vi "PCO_GetTimingStruct.vi"(8 "error in (no error)":errorcluster {"code" format="%x"}, 11 "ph":u64) -> (0 "error out":errorcluster {"code" format="%x"}, 1 "strTiming":T1, 2 "ErrorMessage":i32 format="%x", 3 "ph out":u64)   [LabVIEW 2019, in "SDK.lvlib" / "TimingControl.lvlib"]
doc: "<b>Description:</b>\nTiming related information is queried from the camera and the variables of the PCO_Timing structure are filled with this information. This function is a combined version of the functions which request information about the current settings of timing related parameter. For a detailed description of each parameter see the functions in this chapter.\n\n<b>Supported camera type:</b>\nAll cameras\n\n<b>Descriptor dependency:</b>\nNone"
uses:
  TimingControl.lvlib
  Structures/Structures.lvlib
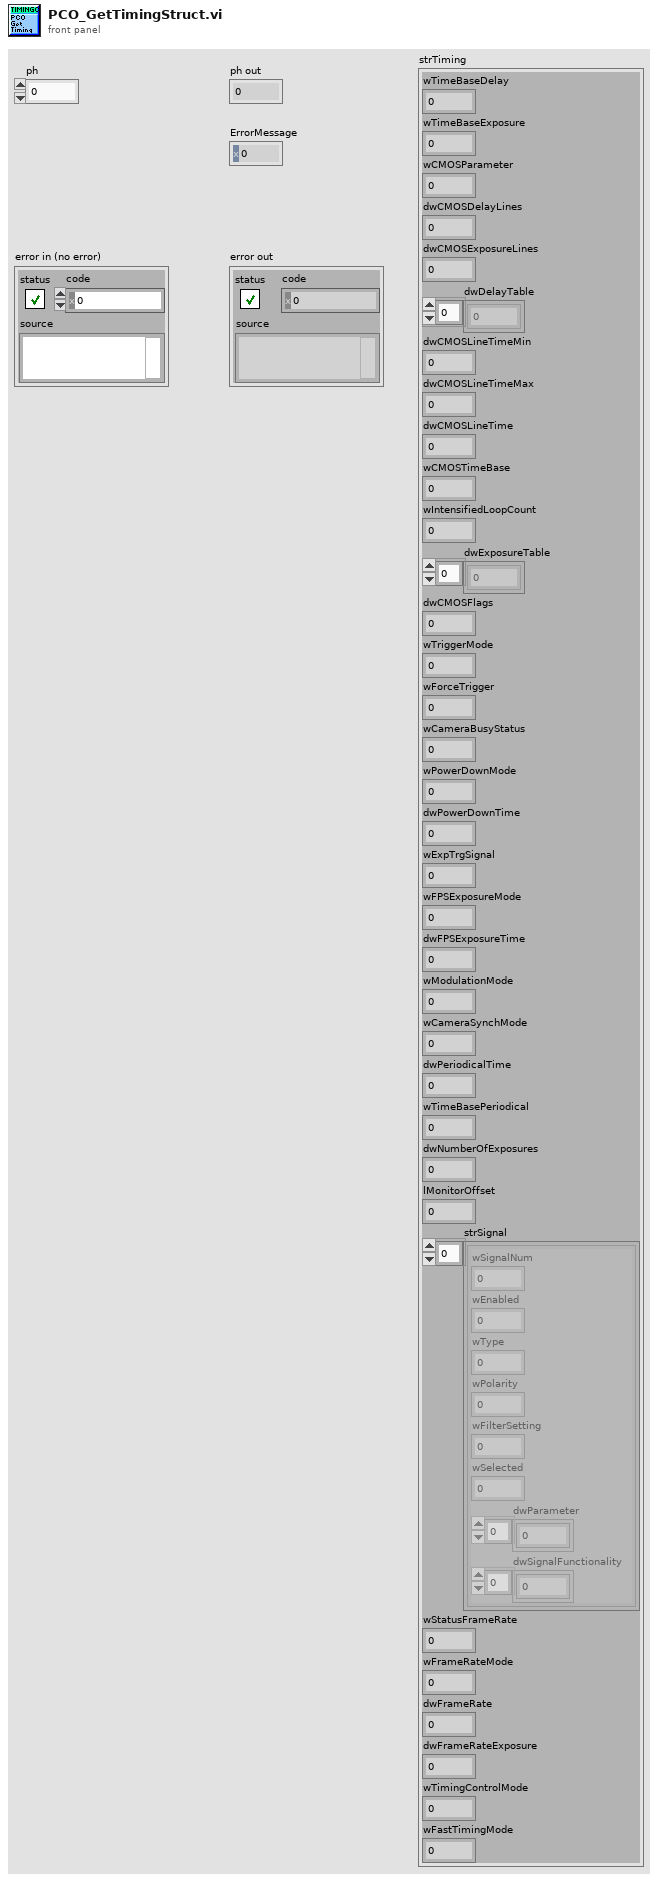
[diagram p1: front panel]
types:
  T1 = cluster{"wTimeBaseDelay":u16, "wTimeBaseExposure":u16, "wCMOSParameter":u16, "dwCMOSDelayLines":u32, "dwCMOSExposureLines":u32, "dwDelayTable":u32[], "dwCMOSLineTimeMin":u32, "dwCMOSLineTimeMax":u32, "dwCMOSLineTime":u32, "wCMOSTimeBase":u16, "wIntensifiedLoopCount":u16, "dwExposureTable":u32[], "dwCMOSFlags":u32, "wTriggerMode":u16, "wForceTrigger":u16, "wCameraBusyStatus":u16, "wPowerDownMode":u16, "dwPowerDownTime":u32, "wExpTrgSignal":u16, "wFPSExposureMode":u16, "dwFPSExposureTime":u32, "wModulationMode":u16, "wCameraSynchMode":u16, "dwPeriodicalTime":u32, "wTimeBasePeriodical":u16, "dwNumberOfExposures":u32, "lMonitorOffset":i32, "strSignal":cluster{"wSignalNum":u16, "wEnabled":u16, "wType":u16, "wPolarity":u16, "wFilterSetting":u16, "wSelected":u16, "dwParameter":u32[], "dwSignalFunctionality":u32[]}[], "wStatusFrameRate":u16, "wFrameRateMode":u16, "dwFrameRate":u32, "dwFrameRateExposure":u32, "wTimingControlMode":u16, "wFastTimingMode":u16}
  T2 = cluster{"wSize":u16, "wTimeBaseDelay":u16, "wTimeBaseExposure":u16, "wCMOSParameter":u16, "dwCMOSDelayLines":u32, "dwCMOSExposureLines":u32, "dwDelayTable":cluster{u32, u32, u32, u32, u32, u32, u32, u32, u32, u32, u32, u32, u32, u32, u32, u32}, "ZZdwDummy1":cluster{"element":u32, "element 2":u32, "element 3":u32, "element 4":u32, "element 5":u32, "element 6":u32, "element 7":u32, "element 8":u32, "element 9":u32, "element 10":u32, "element 11":u32, "element 12":u32, "element 13":u32, "element 14":u32, "element 15":u32, "element 16":u32, "element 17":u32, "element 18":u32, "element 19":u32, "element 20":u32, "element 21":u32, "element 22":u32, "element 23":u32, "element 24":u32, "element 25":u32, "element 26":u32, "element 27":u32, "element 28":u32, "element 29":u32, "element 30":u32, "element 31":u32, "element 32":u32, "element 33":u32, "element 34":u32, "element 35":u32, "element 36":u32, "element 37":u32, "element 38":u32, "element 39":u32, "element 40":u32, "element 41":u32, "element 42":u32, "element 43":u32, "element 44":u32, "element 45":u32, "element 46":u32, "element 47":u32, "element 48":u32, "element 49":u32, "element 50":u32, "element 51":u32, "element 52":u32, "element 53":u32, "element 54":u32, "element 55":u32, "element 56":u32, "element 57":u32, "element 58":u32, "element 59":u32, "element 60":u32, "element 61":u32, "element 62":u32, "element 63":u32, "element 64":u32, "element 65":u32, "element 66":u32, "element 67":u32, "element 68":u32, "element 69":u32, "element 70":u32, "element 71":u32, "element 72":u32, "element 73":u32, "element 74":u32, "element 75":u32, "element 76":u32, "element 77":u32, "element 78":u32, "element 79":u32, "element 80":u32, "element 81":u32, "element 82":u32, "element 83":u32, "element 84":u32, "element 85":u32, "element 86":u32, "element 87":u32, "element 88":u32, "element 89":u32, "element 90":u32, "element 91":u32, "element 92":u32, "element 93":u32, "element 94":u32, "element 95":u32, "element 96":u32, "element 97":u32, "element 98":u32, "element 99":u32, "element 100":u32, "element 101":u32, "element 102":u32, "element 103":u32, "element 104":u32, "element 105":u32, "element 106":u32, "element 107":u32, "element 108":u32, "element 109":u32, "element 110":u32}, "dwCMOSLineTimeMin":u32, "dwCMOSLineTimeMax":u32, "dwCMOSLineTime":u32, "wCMOSTimeBase":u16, "wIntensifiedLoopCount":u16, "dwExposureTable":cluster{u32, u32, u32, u32, u32, u32, u32, u32, u32, u32, u32, u32, u32, u32, u32, u32}, "ZZdwDummy2":cluster{"element":u32, "element 2":u32, "element 3":u32, "element 4":u32, "element 5":u32, "element 6":u32, "element 7":u32, "element 8":u32, "element 9":u32, "element 10":u32, "element 11":u32, "element 12":u32, "element 13":u32, "element 14":u32, "element 15":u32, "element 16":u32, "element 17":u32, "element 18":u32, "element 19":u32, "element 20":u32, "element 21":u32, "element 22":u32, "element 23":u32, "element 24":u32, "element 25":u32, "element 26":u32, "element 27":u32, "element 28":u32, "element 29":u32, "element 30":u32, "element 31":u32, "element 32":u32, "element 33":u32, "element 34":u32, "element 35":u32, "element 36":u32, "element 37":u32, "element 38":u32, "element 39":u32, "element 40":u32, "element 41":u32, "element 42":u32, "element 43":u32, "element 44":u32, "element 45":u32, "element 46":u32, "element 47":u32, "element 48":u32, "element 49":u32, "element 50":u32, "element 51":u32, "element 52":u32, "element 53":u32, "element 54":u32, "element 55":u32, "element 56":u32, "element 57":u32, "element 58":u32, "element 59":u32, "element 60":u32, "element 61":u32, "element 62":u32, "element 63":u32, "element 64":u32, "element 65":u32, "element 66":u32, "element 67":u32, "element 68":u32, "element 69":u32, "element 70":u32, "element 71":u32, "element 72":u32, "element 73":u32, "element 74":u32, "element 75":u32, "element 76":u32, "element 77":u32, "element 78":u32, "element 79":u32, "element 80":u32, "element 81":u32, "element 82":u32, "element 83":u32, "element 84":u32, "element 85":u32, "element 86":u32, "element 87":u32, "element 88":u32, "element 89":u32, "element 90":u32, "element 91":u32, "element 92":u32, "element 93":u32, "element 94":u32, "element 95":u32, "element 96":u32, "element 97":u32, "element 98":u32, "element 99":u32, "element 100":u32, "element 101":u32, "element 102":u32, "element 103":u32, "element 104":u32, "element 105":u32, "element 106":u32, "element 107":u32, "element 108":u32, "element 109":u32, "element 110":u32}, "dwCMOSFlags":u32, "ZZdwDummy3":u32, "wTriggerMode":u16, "wForceTrigger":u16, "wCameraBusyStatus":u16, "wPowerDownMode":u16, "dwPowerDownTime":u32, "wExpTrgSignal":u16, "wFPSExposureMode":u16, "dwFPSExposureTime":u32, "wModulationMode":u16, "wCameraSynchMode":u16, "dwPeriodicalTime":u32, "wTimeBasePeriodical":u16, "ZZwDummy3":u16, "dwNumberOfExposures":u32, "lMonitorOffset":i32, "strSignal":cluster{"PCO_Signal_Raw":cluster{"wSize":u16, "wSignalNum":u16, "wEnabled":u16, "wType":u16, "wPolarity":u16, "wFilterSetting":u16, "wSelected":u16, "ZZwReserved":u16, "dwParameter":cluster{u32, u32, u32, u32}, "dwSignalFunctionality":cluster{u32, u32, u32, u32}, "ZZdwReserved":cluster{u32, u32, u32}}, "PCO_Signal_Raw":cluster{"wSize":u16, "wSignalNum":u16, "wEnabled":u16, "wType":u16, "wPolarity":u16, "wFilterSetting":u16, "wSelected":u16, "ZZwReserved":u16, "dwParameter":cluster{u32, u32, u32, u32}, "dwSignalFunctionality":cluster{u32, u32, u32, u32}, "ZZdwReserved":cluster{u32, u32, u32}}, "PCO_Signal_Raw":cluster{"wSize":u16, "wSignalNum":u16, "wEnabled":u16, "wType":u16, "wPolarity":u16, "wFilterSetting":u16, "wSelected":u16, "ZZwReserved":u16, "dwParameter":cluster{u32, u32, u32, u32}, "dwSignalFunctionality":cluster{u32, u32, u32, u32}, "ZZdwReserved":cluster{u32, u32, u32}}, "PCO_Signal_Raw":cluster{"wSize":u16, "wSignalNum":u16, "wEnabled":u16, "wType":u16, "wPolarity":u16, "wFilterSetting":u16, "wSelected":u16, "ZZwReserved":u16, "dwParameter":cluster{u32, u32, u32, u32}, "dwSignalFunctionality":cluster{u32, u32, u32, u32}, "ZZdwReserved":cluster{u32, u32, u32}}, "PCO_Signal_Raw":cluster{"wSize":u16, "wSignalNum":u16, "wEnabled":u16, "wType":u16, "wPolarity":u16, "wFilterSetting":u16, "wSelected":u16, "ZZwReserved":u16, "dwParameter":cluster{u32, u32, u32, u32}, "dwSignalFunctionality":cluster{u32, u32, u32, u32}, "ZZdwReserved":cluster{u32, u32, u32}}, "PCO_Signal_Raw":cluster{"wSize":u16, "wSignalNum":u16, "wEnabled":u16, "wType":u16, "wPolarity":u16, "wFilterSetting":u16, "wSelected":u16, "ZZwReserved":u16, "dwParameter":cluster{u32, u32, u32, u32}, "dwSignalFunctionality":cluster{u32, u32, u32, u32}, "ZZdwReserved":cluster{u32, u32, u32}}, "PCO_Signal_Raw":cluster{"wSize":u16, "wSignalNum":u16, "wEnabled":u16, "wType":u16, "wPolarity":u16, "wFilterSetting":u16, "wSelected":u16, "ZZwReserved":u16, "dwParameter":cluster{u32, u32, u32, u32}, "dwSignalFunctionality":cluster{u32, u32, u32, u32}, "ZZdwReserved":cluster{u32, u32, u32}}, "PCO_Signal_Raw":cluster{"wSize":u16, "wSignalNum":u16, "wEnabled":u16, "wType":u16, "wPolarity":u16, "wFilterSetting":u16, "wSelected":u16, "ZZwReserved":u16, "dwParameter":cluster{u32, u32, u32, u32}, "dwSignalFunctionality":cluster{u32, u32, u32, u32}, "ZZdwReserved":cluster{u32, u32, u32}}, "PCO_Signal_Raw":cluster{"wSize":u16, "wSignalNum":u16, "wEnabled":u16, "wType":u16, "wPolarity":u16, "wFilterSetting":u16, "wSelected":u16, "ZZwReserved":u16, "dwParameter":cluster{u32, u32, u32, u32}, "dwSignalFunctionality":cluster{u32, u32, u32, u32}, "ZZdwReserved":cluster{u32, u32, u32}}, "PCO_Signal_Raw":cluster{"wSize":u16, "wSignalNum":u16, "wEnabled":u16, "wType":u16, "wPolarity":u16, "wFilterSetting":u16, "wSelected":u16, "ZZwReserved":u16, "dwParameter":cluster{u32, u32, u32, u32}, "dwSignalFunctionality":cluster{u32, u32, u32, u32}, "ZZdwReserved":cluster{u32, u32, u32}}, "PCO_Signal_Raw":cluster{"wSize":u16, "wSignalNum":u16, "wEnabled":u16, "wType":u16, "wPolarity":u16, "wFilterSetting":u16, "wSelected":u16, "ZZwReserved":u16, "dwParameter":cluster{u32, u32, u32, u32}, "dwSignalFunctionality":cluster{u32, u32, u32, u32}, "ZZdwReserved":cluster{u32, u32, u32}}, "PCO_Signal_Raw":cluster{"wSize":u16, "wSignalNum":u16, "wEnabled":u16, "wType":u16, "wPolarity":u16, "wFilterSetting":u16, "wSelected":u16, "ZZwReserved":u16, "dwParameter":cluster{u32, u32, u32, u32}, "dwSignalFunctionality":cluster{u32, u32, u32, u32}, "ZZdwReserved":cluster{u32, u32, u32}}, "PCO_Signal_Raw":cluster{"wSize":u16, "wSignalNum":u16, "wEnabled":u16, "wType":u16, "wPolarity":u16, "wFilterSetting":u16, "wSelected":u16, "ZZwReserved":u16, "dwParameter":cluster{u32, u32, u32, u32}, "dwSignalFunctionality":cluster{u32, u32, u32, u32}, "ZZdwReserved":cluster{u32, u32, u32}}, "PCO_Signal_Raw":cluster{"wSize":u16, "wSignalNum":u16, "wEnabled":u16, "wType":u16, "wPolarity":u16, "wFilterSetting":u16, "wSelected":u16, "ZZwReserved":u16, "dwParameter":cluster{u32, u32, u32, u32}, "dwSignalFunctionality":cluster{u32, u32, u32, u32}, "ZZdwReserved":cluster{u32, u32, u32}}, "PCO_Signal_Raw":cluster{"wSize":u16, "wSignalNum":u16, "wEnabled":u16, "wType":u16, "wPolarity":u16, "wFilterSetting":u16, "wSelected":u16, "ZZwReserved":u16, "dwParameter":cluster{u32, u32, u32, u32}, "dwSignalFunctionality":cluster{u32, u32, u32, u32}, "ZZdwReserved":cluster{u32, u32, u32}}, "PCO_Signal_Raw":cluster{"wSize":u16, "wSignalNum":u16, "wEnabled":u16, "wType":u16, "wPolarity":u16, "wFilterSetting":u16, "wSelected":u16, "ZZwReserved":u16, "dwParameter":cluster{u32, u32, u32, u32}, "dwSignalFunctionality":cluster{u32, u32, u32, u32}, "ZZdwReserved":cluster{u32, u32, u32}}, "PCO_Signal_Raw":cluster{"wSize":u16, "wSignalNum":u16, "wEnabled":u16, "wType":u16, "wPolarity":u16, "wFilterSetting":u16, "wSelected":u16, "ZZwReserved":u16, "dwParameter":cluster{u32, u32, u32, u32}, "dwSignalFunctionality":cluster{u32, u32, u32, u32}, "ZZdwReserved":cluster{u32, u32, u32}}, "PCO_Signal_Raw":cluster{"wSize":u16, "wSignalNum":u16, "wEnabled":u16, "wType":u16, "wPolarity":u16, "wFilterSetting":u16, "wSelected":u16, "ZZwReserved":u16, "dwParameter":cluster{u32, u32, u32, u32}, "dwSignalFunctionality":cluster{u32, u32, u32, u32}, "ZZdwReserved":cluster{u32, u32, u32}}, "PCO_Signal_Raw":cluster{"wSize":u16, "wSignalNum":u16, "wEnabled":u16, "wType":u16, "wPolarity":u16, "wFilterSetting":u16, "wSelected":u16, "ZZwReserved":u16, "dwParameter":cluster{u32, u32, u32, u32}, "dwSignalFunctionality":cluster{u32, u32, u32, u32}, "ZZdwReserved":cluster{u32, u32, u32}}, "PCO_Signal_Raw":cluster{"wSize":u16, "wSignalNum":u16, "wEnabled":u16, "wType":u16, "wPolarity":u16, "wFilterSetting":u16, "wSelected":u16, "ZZwReserved":u16, "dwParameter":cluster{u32, u32, u32, u32}, "dwSignalFunctionality":cluster{u32, u32, u32, u32}, "ZZdwReserved":cluster{u32, u32, u32}}}, "wStatusFrameRate":u16, "wFrameRateMode":u16, "dwFrameRate":u32, "dwFrameRateExposure":u32, "wTimingControlMode":u16, "wFastTimingMode":u16, "ZZwDummy":cluster{"element":u16, "element 2":u16, "element 3":u16, "element 4":u16, "element 5":u16, "element 6":u16, "element 7":u16, "element 8":u16, "element 9":u16, "element 10":u16, "element 11":u16, "element 12":u16, "element 13":u16, "element 14":u16, "element 15":u16, "element 16":u16, "element 17":u16, "element 18":u16, "element 19":u16, "element 20":u16, "element 22":u16, "element 23":u16, "element 24":u16, "element 25":u16}}
  T3 = cluster{u32, u32, u32, u32, u32, u32, u32, u32, u32, u32, u32, u32, u32, u32, u32, u32}
  T4 = cluster{"PCO_Signal_Raw":cluster{"wSize":u16, "wSignalNum":u16, "wEnabled":u16, "wType":u16, "wPolarity":u16, "wFilterSetting":u16, "wSelected":u16, "ZZwReserved":u16, "dwParameter":cluster{u32, u32, u32, u32}, "dwSignalFunctionality":cluster{u32, u32, u32, u32}, "ZZdwReserved":cluster{u32, u32, u32}}, "PCO_Signal_Raw":cluster{"wSize":u16, "wSignalNum":u16, "wEnabled":u16, "wType":u16, "wPolarity":u16, "wFilterSetting":u16, "wSelected":u16, "ZZwReserved":u16, "dwParameter":cluster{u32, u32, u32, u32}, "dwSignalFunctionality":cluster{u32, u32, u32, u32}, "ZZdwReserved":cluster{u32, u32, u32}}, "PCO_Signal_Raw":cluster{"wSize":u16, "wSignalNum":u16, "wEnabled":u16, "wType":u16, "wPolarity":u16, "wFilterSetting":u16, "wSelected":u16, "ZZwReserved":u16, "dwParameter":cluster{u32, u32, u32, u32}, "dwSignalFunctionality":cluster{u32, u32, u32, u32}, "ZZdwReserved":cluster{u32, u32, u32}}, "PCO_Signal_Raw":cluster{"wSize":u16, "wSignalNum":u16, "wEnabled":u16, "wType":u16, "wPolarity":u16, "wFilterSetting":u16, "wSelected":u16, "ZZwReserved":u16, "dwParameter":cluster{u32, u32, u32, u32}, "dwSignalFunctionality":cluster{u32, u32, u32, u32}, "ZZdwReserved":cluster{u32, u32, u32}}, "PCO_Signal_Raw":cluster{"wSize":u16, "wSignalNum":u16, "wEnabled":u16, "wType":u16, "wPolarity":u16, "wFilterSetting":u16, "wSelected":u16, "ZZwReserved":u16, "dwParameter":cluster{u32, u32, u32, u32}, "dwSignalFunctionality":cluster{u32, u32, u32, u32}, "ZZdwReserved":cluster{u32, u32, u32}}, "PCO_Signal_Raw":cluster{"wSize":u16, "wSignalNum":u16, "wEnabled":u16, "wType":u16, "wPolarity":u16, "wFilterSetting":u16, "wSelected":u16, "ZZwReserved":u16, "dwParameter":cluster{u32, u32, u32, u32}, "dwSignalFunctionality":cluster{u32, u32, u32, u32}, "ZZdwReserved":cluster{u32, u32, u32}}, "PCO_Signal_Raw":cluster{"wSize":u16, "wSignalNum":u16, "wEnabled":u16, "wType":u16, "wPolarity":u16, "wFilterSetting":u16, "wSelected":u16, "ZZwReserved":u16, "dwParameter":cluster{u32, u32, u32, u32}, "dwSignalFunctionality":cluster{u32, u32, u32, u32}, "ZZdwReserved":cluster{u32, u32, u32}}, "PCO_Signal_Raw":cluster{"wSize":u16, "wSignalNum":u16, "wEnabled":u16, "wType":u16, "wPolarity":u16, "wFilterSetting":u16, "wSelected":u16, "ZZwReserved":u16, "dwParameter":cluster{u32, u32, u32, u32}, "dwSignalFunctionality":cluster{u32, u32, u32, u32}, "ZZdwReserved":cluster{u32, u32, u32}}, "PCO_Signal_Raw":cluster{"wSize":u16, "wSignalNum":u16, "wEnabled":u16, "wType":u16, "wPolarity":u16, "wFilterSetting":u16, "wSelected":u16, "ZZwReserved":u16, "dwParameter":cluster{u32, u32, u32, u32}, "dwSignalFunctionality":cluster{u32, u32, u32, u32}, "ZZdwReserved":cluster{u32, u32, u32}}, "PCO_Signal_Raw":cluster{"wSize":u16, "wSignalNum":u16, "wEnabled":u16, "wType":u16, "wPolarity":u16, "wFilterSetting":u16, "wSelected":u16, "ZZwReserved":u16, "dwParameter":cluster{u32, u32, u32, u32}, "dwSignalFunctionality":cluster{u32, u32, u32, u32}, "ZZdwReserved":cluster{u32, u32, u32}}, "PCO_Signal_Raw":cluster{"wSize":u16, "wSignalNum":u16, "wEnabled":u16, "wType":u16, "wPolarity":u16, "wFilterSetting":u16, "wSelected":u16, "ZZwReserved":u16, "dwParameter":cluster{u32, u32, u32, u32}, "dwSignalFunctionality":cluster{u32, u32, u32, u32}, "ZZdwReserved":cluster{u32, u32, u32}}, "PCO_Signal_Raw":cluster{"wSize":u16, "wSignalNum":u16, "wEnabled":u16, "wType":u16, "wPolarity":u16, "wFilterSetting":u16, "wSelected":u16, "ZZwReserved":u16, "dwParameter":cluster{u32, u32, u32, u32}, "dwSignalFunctionality":cluster{u32, u32, u32, u32}, "ZZdwReserved":cluster{u32, u32, u32}}, "PCO_Signal_Raw":cluster{"wSize":u16, "wSignalNum":u16, "wEnabled":u16, "wType":u16, "wPolarity":u16, "wFilterSetting":u16, "wSelected":u16, "ZZwReserved":u16, "dwParameter":cluster{u32, u32, u32, u32}, "dwSignalFunctionality":cluster{u32, u32, u32, u32}, "ZZdwReserved":cluster{u32, u32, u32}}, "PCO_Signal_Raw":cluster{"wSize":u16, "wSignalNum":u16, "wEnabled":u16, "wType":u16, "wPolarity":u16, "wFilterSetting":u16, "wSelected":u16, "ZZwReserved":u16, "dwParameter":cluster{u32, u32, u32, u32}, "dwSignalFunctionality":cluster{u32, u32, u32, u32}, "ZZdwReserved":cluster{u32, u32, u32}}, "PCO_Signal_Raw":cluster{"wSize":u16, "wSignalNum":u16, "wEnabled":u16, "wType":u16, "wPolarity":u16, "wFilterSetting":u16, "wSelected":u16, "ZZwReserved":u16, "dwParameter":cluster{u32, u32, u32, u32}, "dwSignalFunctionality":cluster{u32, u32, u32, u32}, "ZZdwReserved":cluster{u32, u32, u32}}, "PCO_Signal_Raw":cluster{"wSize":u16, "wSignalNum":u16, "wEnabled":u16, "wType":u16, "wPolarity":u16, "wFilterSetting":u16, "wSelected":u16, "ZZwReserved":u16, "dwParameter":cluster{u32, u32, u32, u32}, "dwSignalFunctionality":cluster{u32, u32, u32, u32}, "ZZdwReserved":cluster{u32, u32, u32}}, "PCO_Signal_Raw":cluster{"wSize":u16, "wSignalNum":u16, "wEnabled":u16, "wType":u16, "wPolarity":u16, "wFilterSetting":u16, "wSelected":u16, "ZZwReserved":u16, "dwParameter":cluster{u32, u32, u32, u32}, "dwSignalFunctionality":cluster{u32, u32, u32, u32}, "ZZdwReserved":cluster{u32, u32, u32}}, "PCO_Signal_Raw":cluster{"wSize":u16, "wSignalNum":u16, "wEnabled":u16, "wType":u16, "wPolarity":u16, "wFilterSetting":u16, "wSelected":u16, "ZZwReserved":u16, "dwParameter":cluster{u32, u32, u32, u32}, "dwSignalFunctionality":cluster{u32, u32, u32, u32}, "ZZdwReserved":cluster{u32, u32, u32}}, "PCO_Signal_Raw":cluster{"wSize":u16, "wSignalNum":u16, "wEnabled":u16, "wType":u16, "wPolarity":u16, "wFilterSetting":u16, "wSelected":u16, "ZZwReserved":u16, "dwParameter":cluster{u32, u32, u32, u32}, "dwSignalFunctionality":cluster{u32, u32, u32, u32}, "ZZdwReserved":cluster{u32, u32, u32}}, "PCO_Signal_Raw":cluster{"wSize":u16, "wSignalNum":u16, "wEnabled":u16, "wType":u16, "wPolarity":u16, "wFilterSetting":u16, "wSelected":u16, "ZZwReserved":u16, "dwParameter":cluster{u32, u32, u32, u32}, "dwSignalFunctionality":cluster{u32, u32, u32, u32}, "ZZdwReserved":cluster{u32, u32, u32}}}
  T5 = cluster{"wSignalNum":u16, "wEnabled":u16, "wType":u16, "wPolarity":u16, "wFilterSetting":u16, "wSelected":u16, "dwParameter":u32[], "dwSignalFunctionality":u32[]}
  T6 = cluster{"wSignalNum":u16, "wEnabled":u16, "wType":u16, "wPolarity":u16, "wFilterSetting":u16, "wSelected":u16, "dwParameter":u32[], "dwSignalFunctionality":u32[]}[]
  T7 = cluster{"wSize":u16, "wSignalNum":u16, "wEnabled":u16, "wType":u16, "wPolarity":u16, "wFilterSetting":u16, "wSelected":u16, "ZZwReserved":u16, "dwParameter":cluster{u32, u32, u32, u32}, "dwSignalFunctionality":cluster{u32, u32, u32, u32}, "ZZdwReserved":cluster{u32, u32, u32}}[]
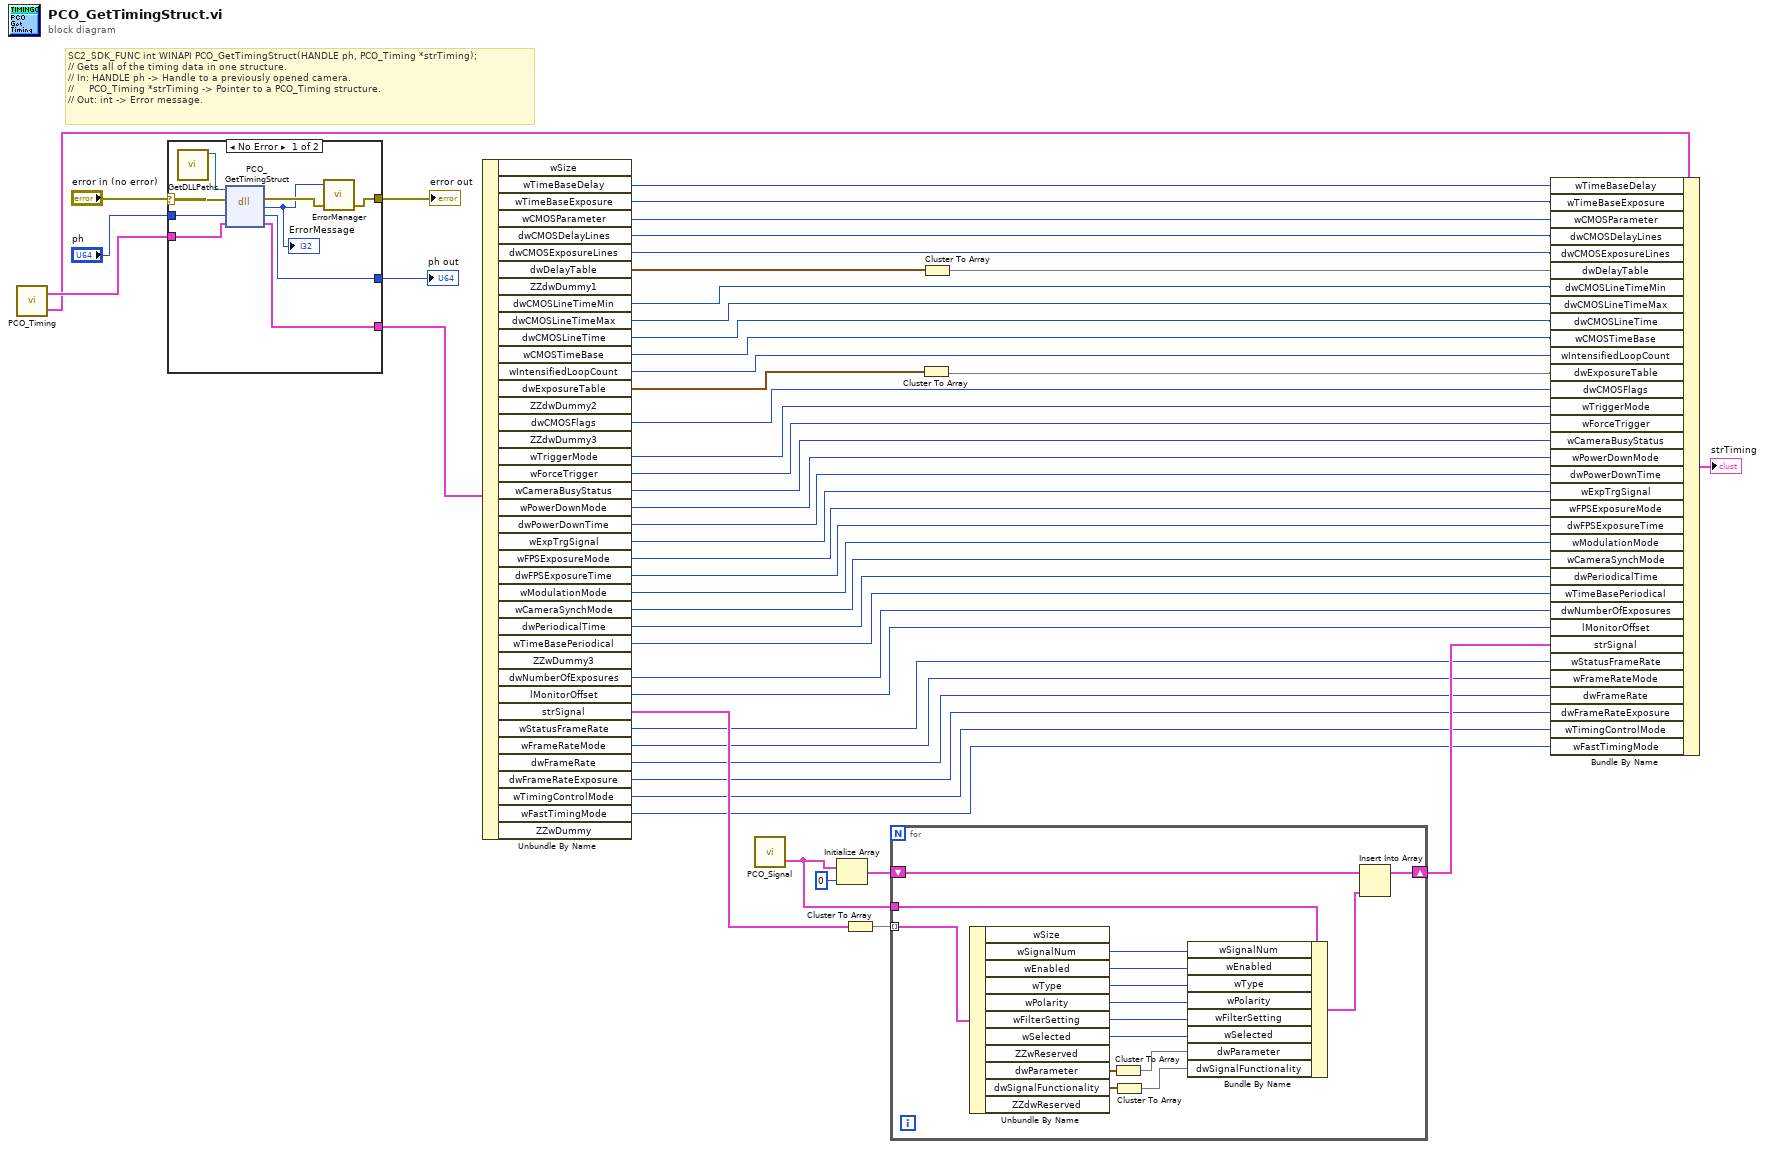
[diagram p0: block diagram]
diagram:
  # "SC2_SDK_FUNC int WINAPI PCO_GetTimingStruct(HANDLE ph, PCO_Timing *strTiming);\n// Gets all of the timing data in one structure.\n// In: HANDLE ph -> Handle to a previously opened camera.\n//     PCO_Timing *strTiming -> Pointer to a PCO_Timing structure.\n// Out: int -> Error message."
  n1 = call "PCO_Timing.vi"() -> ("PCO_Timing"=w36:T1, "PCO_Timing_Raw"=w38:T2)  [unwired: 4 in, 2 out]
  n2 = case shown="No Error" "error in (no error)" {
    selector: "error in (no error)" -> [w54 w61]
    tunnel: "ph" -> [w58 w60]
    tunnel: [w57 w60] -> w48
    tunnel: w38 -> [w56 w59]
    tunnel: [w55 w59] -> w41
    tunnel: [w52 w61] -> w47
    frame No Error {
      n3 = call "GetDLLPaths.vi"() -> ("SC2_Cam_Path"=w50:path)  [unwired: 9 in, 2 out]
      n4 = dll-call lib="?" fn="PCO_GetTimingStruct"(path in=w50, error in=w54, "ph"=w58, "strTiming"=w56) -> (error out=w53:errorcluster, "return type"=w51:i32, "ph"=w57:u64, "strTiming"=w55:T2)  [unwired: 1 in, 1 out]
      "ErrorMessage" <- w51
      n5 = call "ErrorManager.vi"("error in (no error)"=w53, "error code"=w51) -> ("error out"=w52:errorcluster)  [unwired: 3 in]
    }
    frame Error {
    }
  }
  "ph out" <- w48
  "error out" <- w47
  n6 = Unbundle By Name(w41) -> ("wTimeBaseDelay"=w33:u16, "wTimeBaseExposure"=w32:u16, "wCMOSParameter"=w31:u16, "dwCMOSDelayLines"=w30:u32, "dwCMOSExposureLines"=w29:u32, "dwDelayTable"=w40:T3, "dwCMOSLineTimeMin"=w27:u32, "dwCMOSLineTimeMax"=w26:u32, "dwCMOSLineTime"=w25:u32, "wCMOSTimeBase"=w24:u16, "wIntensifiedLoopCount"=w34:u16, "dwExposureTable"=w39:T3, "dwCMOSFlags"=w23:u32, "wTriggerMode"=w22:u16, "wForceTrigger"=w21:u16, "wCameraBusyStatus"=w20:u16, "wPowerDownMode"=w19:u16, "dwPowerDownTime"=w18:u32, "wExpTrgSignal"=w17:u16, "wFPSExposureMode"=w16:u16, "dwFPSExposureTime"=w15:u32, "wModulationMode"=w14:u16, "wCameraSynchMode"=w13:u16, "dwPeriodicalTime"=w12:u32, "wTimeBasePeriodical"=w11:u16, "dwNumberOfExposures"=w10:u32, "lMonitorOffset"=w9:i32, "strSignal"=w37:T4, "wStatusFrameRate"=w7:u16, "wFrameRateMode"=w6:u16, "dwFrameRate"=w5:u32, "dwFrameRateExposure"=w4:u32, "wTimingControlMode"=w3:u16, "wFastTimingMode"=w2:u16)  [unwired: 6 out]
  n7 = call "PCO_Signal.vi"() -> ("PCO_Signal"=w42:T5)  [unwired: 4 in, 3 out]
  n8 = Initialize Array(w42, 0 ("dimension size")) -> (w43:T6)
  n9 = Cluster To Array(cluster=w37) -> (array=w45:T7)
  n10 = for {
    tunnel: w45 -> [w74] mode=indexing
    shift-right: [w76] -> w8
    shift-left: w43 -> [w75]
    tunnel: w42 -> [w73]
    n11 = Unbundle By Name(w74) -> ("wSignalNum"=w72:u16, "wEnabled"=w71:u16, "wType"=w70:u16, "wPolarity"=w69:u16, "wFilterSetting"=w68:u16, "wSelected"=w67:u16, "dwParameter"=w66:cluster{u32, u32, u32, u32}, "dwSignalFunctionality"=w63:cluster{u32, u32, u32, u32})  [unwired: 3 out]
    n12 = Cluster To Array(cluster=w66) -> (array=w65:u32[])
    n13 = Cluster To Array(cluster=w63) -> (array=w64:u32[])
    n14 = Bundle By Name(cluster=w73, "wSignalNum"=w72, "wEnabled"=w71, "wType"=w70, "wPolarity"=w69, "wFilterSetting"=w68, "wSelected"=w67, "dwParameter"=w65, "dwSignalFunctionality"=w64) -> (w62:T5)
    n15 = Insert Into Array(array=w75, new element=w62) -> (w76:T6)  [unwired: 1 in]
  }
  n16 = Cluster To Array(cluster=w39) -> (array=w35:u32[])
  n17 = Cluster To Array(cluster=w40) -> (array=w28:u32[])
  n18 = Bundle By Name(cluster=w36, "wTimeBaseDelay"=w33, "wTimeBaseExposure"=w32, "wCMOSParameter"=w31, "dwCMOSDelayLines"=w30, "dwCMOSExposureLines"=w29, "dwDelayTable"=w28, "dwCMOSLineTimeMin"=w27, "dwCMOSLineTimeMax"=w26, "dwCMOSLineTime"=w25, "wCMOSTimeBase"=w24, "wIntensifiedLoopCount"=w34, "dwExposureTable"=w35, "dwCMOSFlags"=w23, "wTriggerMode"=w22, "wForceTrigger"=w21, "wCameraBusyStatus"=w20, "wPowerDownMode"=w19, "dwPowerDownTime"=w18, "wExpTrgSignal"=w17, "wFPSExposureMode"=w16, "dwFPSExposureTime"=w15, "wModulationMode"=w14, "wCameraSynchMode"=w13, "dwPeriodicalTime"=w12, "wTimeBasePeriodical"=w11, "dwNumberOfExposures"=w10, "lMonitorOffset"=w9, "strSignal"=w8, "wStatusFrameRate"=w7, "wFrameRateMode"=w6, "dwFrameRate"=w5, "dwFrameRateExposure"=w4, "wTimingControlMode"=w3, "wFastTimingMode"=w2) -> (→"strTiming":T1)
